vi "Generate R(x,alpha).vi"(1 "Axis":enum16{"x", "y", "z"}(ring), 3 "Angle (degrees)":dbl format="%.2f") -> (0 "Final Frame":T1={"nx"=1.0, "ny"=0.0, "nz"=0.0, "nw"=0.0, "ox"=0.0, "oy"=0.72, "oz"=0.72, "ow"=0.0, "ax"=0.0, "ay"=-0.72, "az"=0.72, "aw"=0.0, "Px"=5.0, "Py"=-0.72, "Pz"=3.5999999999999996, "Pw"=1.0} {"Pw" format="%.2f"; "Pz" format="%.2f"; "Py" format="%.2f"; "Px" format="%.2f"; "aw" format="%.2f"; "az" format="%.2f"; "ay" format="%.2f"; "ax" format="%.2f"; "ow" format="%.2f"; "nw" format="%.2f"; "oz" format="%.2f"; "oy" format="%.2f"; "ox" format="%.2f"; "nz" format="%.2f"; "ny" format="%.2f"; "nx" format="%.2f"})   [LabVIEW 2010]
uses:
  ReferenceFrame.ctl
panel:
  in  "Default":T1={"nx"=1.0, "ny"=0.0, "nz"=0.0, "nw"=0.0, "ox"=0.0, "oy"=1.0, "oz"=0.0, "ow"=0.0, "ax"=0.0, "ay"=0.0, "az"=1.0, "aw"=0.0, "Px"=0.0, "Py"=0.0, "Pz"=0.0, "Pw"=1.0} {"Pw" format="%.2f"; "Pz" format="%.2f"; "Py" format="%.2f"; "Px" format="%.2f"; "aw" format="%.2f"; "az" format="%.2f"; "ay" format="%.2f"; "ax" format="%.2f"; "ow" format="%.2f"; "nw" format="%.2f"; "oz" format="%.2f"; "oy" format="%.2f"; "ox" format="%.2f"; "nz" format="%.2f"; "ny" format="%.2f"; "nx" format="%.2f"}
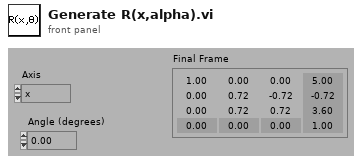
[diagram p1: front panel]
types:
  T1 = typedef "ReferenceFrame.ctl" = cluster{"nx":dbl, "ny":dbl, "nz":dbl, "nw":dbl, "ox":dbl, "oy":dbl, "oz":dbl, "ow":dbl, "ax":dbl, "ay":dbl, "az":dbl, "aw":dbl, "Px":dbl, "Py":dbl, "Pz":dbl, "Pw":dbl}
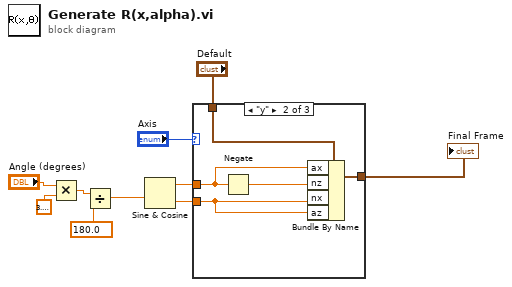
[diagram p0: block diagram]
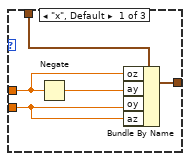
[diagram p2: hidden frame]
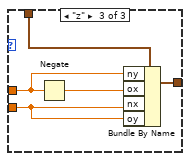
[diagram p3: hidden frame]
diagram:
  n1 = Multiply(x="Angle (degrees)", y=3.141592653589793) -> (x*y=w8:dbl)
  n2 = Divide(x=w8, y=180.0) -> (x/y=w3:dbl)
  n3 = Sine & Cosine(0:w3) -> (1:w1:dbl, 2:w2:dbl)
  n4 = case shown="\"y\"" "Axis" {
    tunnel: "Default" -> [w15 w20 w25]
    tunnel: [w14 w19 w24] -> w4
    tunnel: w2 -> [w11 w16 w21]
    tunnel: w1 -> [w12 w17 w22]
    frame "x", Default {
      n5 = Negate(x=w12) -> (-x=w13:dbl)
      n6 = Bundle By Name(cluster=w15, "oz"=w12, "ay"=w13, "oy"=w11, "az"=w11) -> (w14:T1)
    }
    frame "y" {
      n7 = Negate(x=w17) -> (-x=w18:dbl)
      n8 = Bundle By Name(cluster=w20, "ax"=w17, "nz"=w18, "nx"=w16, "az"=w16) -> (w19:T1)
    }
    frame "z" {
      n9 = Negate(x=w22) -> (-x=w23:dbl)
      n10 = Bundle By Name(cluster=w25, "ny"=w22, "ox"=w23, "nx"=w21, "oy"=w21) -> (w24:T1)
    }
  }
  "Final Frame" <- w4
